vi "Read Attributes.vi"(11 "New Message Msg":refnum<class "New Message Msg.lvclass">) -> (2 "Payload":cluster{"New Message":string})   [LabVIEW 2017, in "WebSocket Client.lvlib" / "New Message Msg.lvclass"]
uses:
  New Message Msg.lvclass
  New Message Msg.lvclass/New Message Msg.ctl
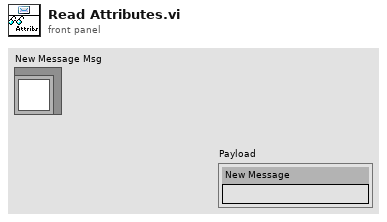
[diagram p1: front panel]
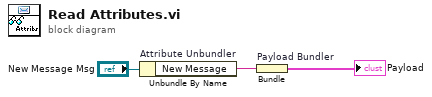
[diagram p0: block diagram]
diagram:
  n1 = Unbundle By Name "Attribute Unbundler"("New Message Msg") -> ("New Message"=w1:string)
  n2 = Bundle "Payload Bundler"("New Message"=w1) -> (→"Payload":cluster{"New Message":string})  [unwired: 1 in]
